vi "calculate phase shift bytes.vi"(8 "start2 - start1":u16 step=5, 9 "width2":u16=37 max=180 step=5, 10 "width1":u16=37 max=180 step=5, 11 "overall phase shift (deg)":u16 step=5) -> (3 "phase shifts":u8[](array[numeric]))   [LabVIEW 2017]
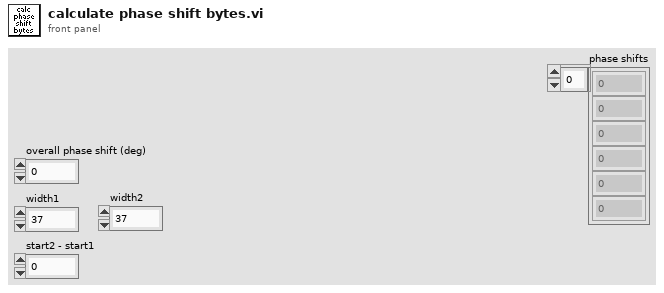
[diagram p1: front panel]
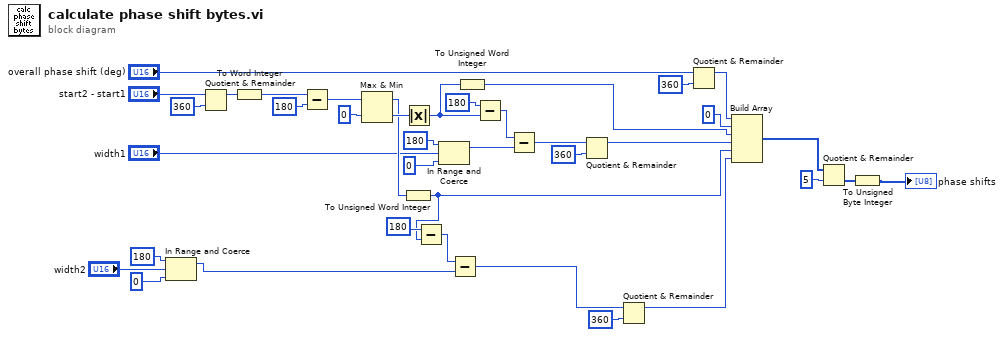
[diagram p0: block diagram]
diagram:
  n1 = In Range and Coerce(upper limit=u16 180, x="width2", lower limit=u16 0) -> (coerced(x)=w7:u16)  [unwired: 1 out]
  n2 = Quotient & Remainder(x="start2 - start1", y=u16 360) -> (x-y*floor(x/y)=w12:u16)  [unwired: 1 out]
  n3 = To Word Integer(number=w12) -> (16bit integer=w36:i16)
  n4 = Subtract(x=w36, y=i16 180) -> (x-y=w35:i16)
  n5 = Max & Min(x=w35, y=i16 0) -> (max(x,y)=w30:i16, min(x,y)=w32:i16)
  n6 = To Unsigned Word Integer(number=w30) -> (unsigned 16bit integer=w8:u16)
  n7 = Absolute Value(x=w32) -> (abs(x)=w17:i16)
  n8 = Subtract(x=u16 180 ("upper limit"), y=w8) -> (x-y=w10:u16)
  n9 = In Range and Coerce(upper limit=u16 180, x="width1", lower limit=u16 0) -> (coerced(x)=w15:u16)  [unwired: 1 out]
  n10 = Subtract(x=w10, y=w7) -> (x-y=w5:u16)
  n11 = To Unsigned Word Integer(number=w17) -> (unsigned 16bit integer=w31:u16)
  n12 = Subtract(x=u16 180 ("upper limit"), y=w17) -> (x-y=w16:u16)
  n13 = Subtract(x=w16, y=w15) -> (x-y=w13:u16)
  n14 = Quotient & Remainder(x=w13, y=u16 360) -> (x-y*floor(x/y)=w11:u16)  [unwired: 1 out]
  n15 = Quotient & Remainder(x=w5, y=u16 360) -> (x-y*floor(x/y)=w4:u16)  [unwired: 1 out]
  n16 = Quotient & Remainder(x="overall phase shift (deg)", y=u16 360) -> (x-y*floor(x/y)=w25:u16)  [unwired: 1 out]
  n17 = Build Array(w25, u16 0 ("element"), w31, w11, w8, w4) -> (w3:u16[])
  n18 = Quotient & Remainder(x=w3, y=u8 5) -> (floor(x/y)=w2:u16[])  [unwired: 1 out]
  n19 = To Unsigned Byte Integer(number=w2) -> (unsigned 8bit integer=→"phase shifts":u8[])
